vi "Decompose Map - Variant Map Value - Decomposes Successfully.vi"() -> ()   [LabVIEW 2019]
uses:
  <vilib>/addons/_JKI Toolkits/Caraya/classes/Assert/Assert Equal Value_Variant.vi
  Composition/Composition.lvlib
  <vilib>/addons/_JKI Toolkits/Caraya/classes/Test/Test.lvclass
  <vilib>/addons/_JKI Toolkits/Caraya/classes/Assert/Assert.lvclass
panel:
  out "error out":errorcluster
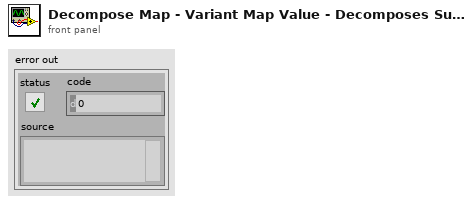
[diagram p1: front panel]
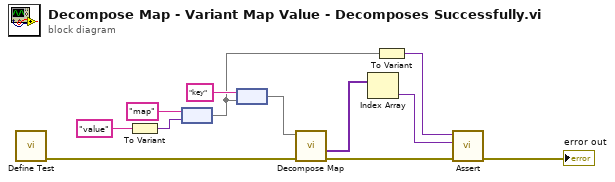
[diagram p0: block diagram]
diagram:
  n1 = call <vilib>:"Define Test.vi"() -> ("error out"=w7:errorcluster)  [unwired: 10 in, 1 out]
  n2 = To Variant(anything="value" ("key")) -> (Variant=w2:variant)
  n3 = node("map" ("key"), w2) -> (w1:map{string, variant})
  n4 = node("key" ("key"), w1) -> (w6:map{string, map{string, variant}})
  n5 = call "Decompose Map.vi"("error in (no error)"=w7, "Variant Map"=w6) -> ("error out"=w11:errorcluster, "Values"=w5:variant[])  [unwired: 6 in, 2 out]
  n6 = Index Array(array=w5) -> (element=w10:variant)  [unwired: 1 in]
  n7 = To Variant(anything=w1) -> (Variant=w4:variant)
  n8 = call-poly <vilib>:"Assert.vi"("error in (no error)"=w11, "Y"=w10, "X"=w4) -> ("error out"=→"error out":errorcluster)  [unwired: 7 in, 1 out]
